vi "CreateTextObjects.vi"(0 "reference in":refnum<class "Control.lvclass">, 2 "VI Name":string, 5 "error in (no error)":errorcluster) -> (14 "reference out":refnum<class "Control.lvclass">, 15 "HTML":string, 19 "error out":errorcluster)   [LabVIEW 2014, in "Control.lvclass"]
uses:
  Control.lvclass
  Text_class/Text.lvclass
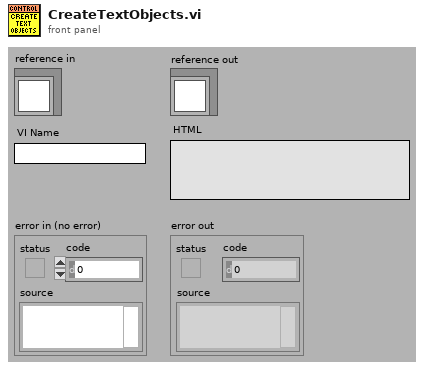
[diagram p1: front panel]
types:
  T1 = typedef "Control.lvclass/Attributes.ctl" = cluster{"Description":string, "Indicator":bool, "Default Value":variant, "Control Index":i32, "Label":refnum<class "Text.lvclass">, "Caption":refnum<class "Text.lvclass">, "Use Picture":bool, "Image 1":T2, "Image 2":T2}
  T2 = typedef "imagedata.ctl" = cluster{"image type":i32, "image depth":i32, "image":u8[], "mask":u8[], "colors":u32[], "Rectangle":cluster{"left":i16, "top":i16, "right":i16, "bottom":i16}}
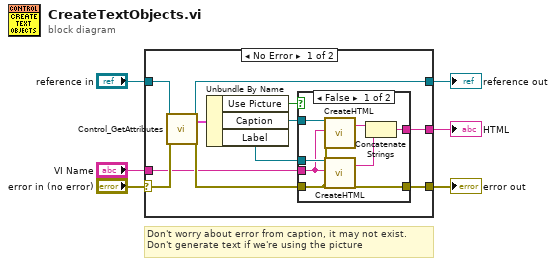
[diagram p0: block diagram]
diagram:
  # "Don't worry about error from caption, it may not exist.\nDon't generate text if we're using the picture"
  n1 = case shown="No Error" "error in (no error)" {
    selector: "error in (no error)" -> [w17 w28]
    tunnel: [w15 w28] -> w5
    tunnel: [w12 w27] -> w3
    tunnel: "reference in" -> [w13 w27]
    tunnel: [w9 _] -> w2
    tunnel: "VI Name" -> [w8 _]
    frame No Error {
      n2 = call "Control_GetAttributes.vi"("reference in"=w13, "error in (no error)"=w17) -> ("reference out"=w12:refnum<class "Control.lvclass">, "Data"=w14:T1, "error out"=w16:errorcluster)  [unwired: 14 in, 1 out]
      n3 = Unbundle By Name(w14) -> ("Use Picture"=w7:bool, "Caption"=w11:refnum<class "Text.lvclass">, "Label"=w10:refnum<class "Text.lvclass">)
      n4 = case shown="False" w7 {
        tunnel: w16 -> [w25 w26]
        tunnel: [w24 w26] -> w15
        tunnel: w11 -> [w23 _]
        tunnel: w10 -> [w22 _]
        tunnel: [w19 _] -> w9
        tunnel: w8 -> [w18 _]
        frame False {
          n5 = call-dynamic "CreateHTML.vi"("reference in"=w23, "VI Name"=w18, "error in (no error)"=w25) -> ("HTML"=w21:string)  [unwired: 10 in, 6 out]
          n6 = call-dynamic "CreateHTML.vi"("reference in"=w22, "VI Name"=w18, "error in (no error)"=w25) -> ("HTML"=w20:string, "error out"=w24:errorcluster)  [unwired: 10 in, 5 out]
          n7 = Concatenate Strings(w21, w20) -> (w19:string)
        }
        frame True {
        }
      }
    }
    frame Error {
    }
  }
  "error out" <- w5
  "reference out" <- w3
  "HTML" <- w2
